vi "niHWS Set Wfm Attribute.vi"   [LabVIEW 2013]
doc: "Sets a particular attribute of a waveform."
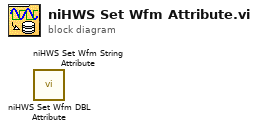
[diagram p0: block diagram]
diagram:
  n1 = call "niHWS Set Wfm DBL Attribute.vi"() -> ()  [unwired: 10 in, 2 out]
  n2 = call "niHWS Set Wfm String Attribute.vi"() -> ()  [unwired: 10 in, 2 out]
